vi "Actor Core.vi"(8 "error in":errorcluster, 11 "Nested in":refnum<class "SCLB_Template.lvclass">) -> (0 "error out":errorcluster, 3 "Actor out":refnum<class "Actor.lvclass">)   [LabVIEW 2021, in "SCLB_Template.lvclass"]
doc: "(<B>Filename</B>: Actor Framework.lvlib:Actor.lvclass:Actor Core.vi)\n\nReceives messages to the actor, reacts to them, and initiates any error handling that may shut the actor down.\n\nDescendant classes may override this VI to append parallel tasks for the actor to complete while it handles messages. Overrides use the Call Parent Method node."
uses:
  SCLB_Template.lvclass
  C:/Program Files (x86)/National Instruments/LabVIEW 2021/user.lib/John_Lib/AbstractActorTemplate/AbstractActorTemplate/UIActorTop.lvclass
  C:/Program Files (x86)/National Instruments/LabVIEW 2021/vi.lib/ActorFramework/Actor/Actor.lvclass
  <vilib>/ActorFramework/Actor/Actor.lvclass
  <userlib>/John_Lib/Control_Lib/SCLB_Lib/SCLB_Lib.lvclass
  SCLB_Template.lvclass/SCLB_Template.ctl
  <vilib>/ActorFramework/Actor/Actor.lvclass/Actor.ctl
  <vilib>/ActorFramework/Message Enqueuer/Message Enqueuer.lvclass/Message Enqueuer.ctl
  <vilib>/ActorFramework/Message Enqueuer/Init from Existing Queue.vi
  <vilib>/ActorFramework/Message Enqueuer/Enqueue.vi
  <userlib>/John_Lib/AbstractActorTemplate/UIActorTop Messages/UI Initialize Msg/UI Initialize Msg.lvclass
  C:/Program Files (x86)/National Instruments/LabVIEW 2021/vi.lib/ActorFramework/Message/Message.lvclass
  <vilib>/ActorFramework/Stop Msg/Stop Msg.lvclass
  <vilib>/ActorFramework/Message Priority Queue/Priority Enqueue.vi
  <vilib>/ActorFramework/Message Enqueuer/Message Enqueuer.lvclass
  <userlib>/John_Lib/AbstractActorTemplate/AbstractActorTemplate/UIActorTop.lvclass
panel:
  in  "Menu_Listbox":i32(listbox)
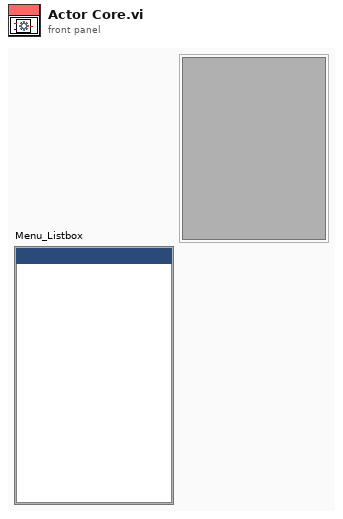
[diagram p1: front panel]
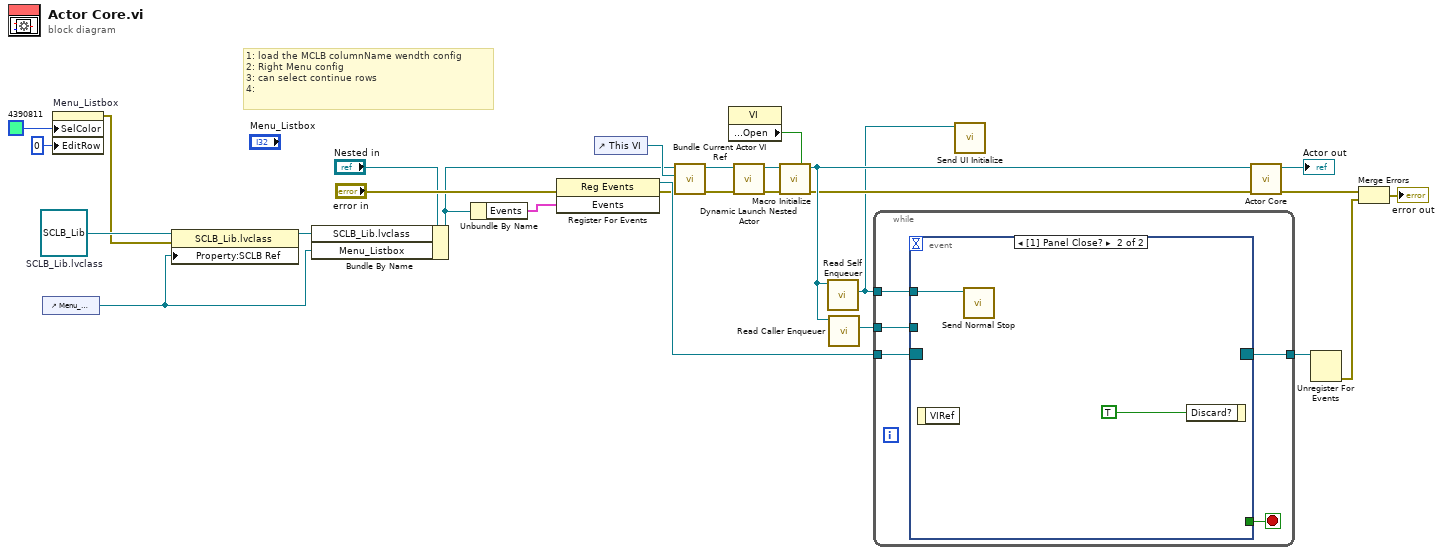
[diagram p0: block diagram]
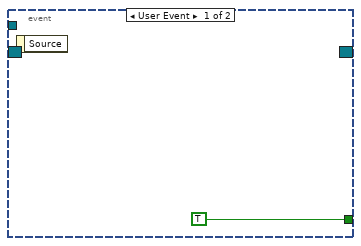
[diagram p2: hidden frame]
diagram:
  w6 = refnum<class "SCLB_Lib.lvclass"> refnum  # SCLB_Lib.lvclass
  # "1: load the MCLB columnName wendth config\n2: Right Menu config\n3: can select continue rows\n4:"
  n1 = control-ref of="Menu_Listbox"() -> (w5:refnum<vi>)
  n2 = property on="Menu_Listbox" class="LstBox (strict)"("SelColor"=u32 4390811 ("OK"), "EditRow"=0 ("Edit Row")) -> (error out=w2:errorcluster)  [unwired: 2 in, 1 out]
  n3 = property class="SCLB_Lib.lvclass"(reference=w6, error in=w2, "Property:SCLB Ref"=w5) -> (reference out=w7:refnum<class "SCLB_Lib.lvclass">)  [unwired: 1 out]
  n4 = Bundle By Name(cluster="Nested in", "SCLB_Lib.lvclass"=w7, "Menu_Listbox"=w5) -> (w8:refnum<class "SCLB_Template.lvclass">)
  n5 = Unbundle By Name(w8) -> ("Events"=w25:cluster{"Stop":refnum<user-event>})
  n6 = register-events ("Main Register for Events")(error in="error in", w25) -> (reference out=w26:refnum<event-registration>, error out=w11:errorcluster)  [unwired: 1 in]
  n7 = control-ref of="This VI"() -> (w9:refnum<vi>)
  n8 = call <userlib>:"Bundle Current Actor VI Ref.vi"("error in (no error)"=w11, "This VI"=w9, "UI ActorTop in"=w8) -> ("error out"=w10:errorcluster, "UI ActorTop out"=w12:refnum<class "SCLB_Template.lvclass">)  [unwired: 5 in, 2 out]
  n9 = property class="VI"() -> ("Front Panel.Open"=w21:bool)  [unwired: 2 in, 2 out]
  n10 = call-dynamic "Dynamic Launch Nested Actor.vi"("error in (no error)"=w10, "UI ActorTop in"=w12) -> ("error out"=w22:errorcluster, "UI ActorTop out"=w23:refnum<class "SCLB_Template.lvclass">)  [unwired: 8 in]
  n11 = call-dynamic "Macro Initialize.vi"("Front Panel Window:Open"=w21, "error in (no error)"=w22, "UI ActorTop in"=w23) -> ("error out"=w15:errorcluster, "UI ActorTop out"=w19:refnum<class "SCLB_Template.lvclass">)  [unwired: 7 in]
  n12 = call <vilib>:"Read Self Enqueuer.vi"("Actor"=w19) -> ("Self Enqueuer"=w1:refnum<class "Message Enqueuer.lvclass">)  [unwired: 10 in]
  n13 = call <vilib>:"Read Caller Enqueuer.vi"("Actor"=w19) -> ("Caller Enqueuer"=w14:refnum<class "Message Enqueuer.lvclass">)  [unwired: 10 in]
  n14 = while {
    tunnel: w26 -> [w32]
    tunnel: [w30] -> w24
    tunnel: w1 -> [w29]
    tunnel: w14 -> [w28]
    stop <- w31 stop-if-true
    n15 = event "UI Events" shown="[1] Panel Close?" {
      selector: w32 -> [_ _]
      dyn-events: [_ _] -> w30
      timeout: _ -> [_ _]
      tunnel: [TRUE _] -> w31
      tunnel: w29 -> [_ w34]
      tunnel: w28 -> [_ _]
      event User Event {
        n16 = event-data() -> ()  [unwired: 1 in, 1 out]
      }
      event Panel Close? {
        n17 = event-data() -> ()  [unwired: 1 in, 1 out]
        n18 = call <vilib>:"Send Normal Stop.vi"("Message Enqueuer"=w34) -> ()  [unwired: 10 in, 1 out]
        n19 = event-data("Discard?"=TRUE) -> ()  [unwired: 1 in, 1 out]
      }
    }
  }
  n20 = call <userlib>:"Send UI Initialize.vi"("Message Enqueuer"=w1) -> ()  [unwired: 9 in, 2 out]
  n21 = call-parent "Actor Core.vi"("error in"=w15, "Actor in"=w19) -> ("error out"=w17:errorcluster, "Actor out"=→"Actor out":refnum<class "Actor.lvclass">)  [unwired: 8 in]
  n22 = Unregister For Events(event registration refnum=w24) -> (error out=w18:errorcluster)  [unwired: 1 in]
  n23 = Merge Errors(w17, w18) -> (→"error out":errorcluster)
